vi "Write Stop Position.vi"(8 "error in (no error)":errorcluster, 10 "Stop Position":u32, 11 "Video File in":refnum<class "Video File.lvclass">) -> (0 "error out":errorcluster, 3 "Video File out":refnum<class "Video File.lvclass">)   [LabVIEW 2018, in "Video File.lvclass"]
uses:
  Video File.lvclass
  Video File.lvclass/Video File.ctl
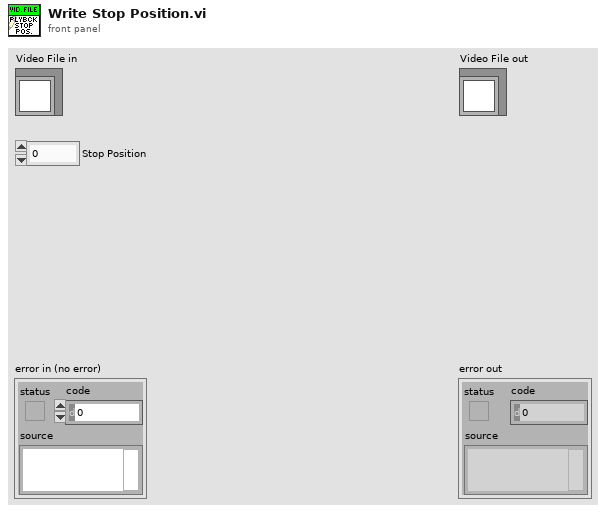
[diagram p1: front panel]
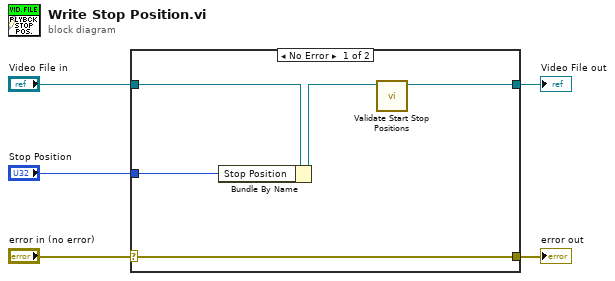
[diagram p0: block diagram]
diagram:
  n1 = case shown="No Error" "error in (no error)" {
    selector: "error in (no error)" -> [w10 w11]
    tunnel: [w10 w11] -> w4
    tunnel: [w6 w12] -> w2
    tunnel: "Video File in" -> [w9 w12]
    tunnel: "Stop Position" -> [w8 _]
    frame No Error {
      n2 = Bundle By Name(cluster=w9, "Stop Position"=w8) -> (w7:refnum<class "Video File.lvclass">)
      n3 = call-dynamic "Validate Start Stop Positions.vi"("Video File in"=w7) -> ("Video File out"=w6:refnum<class "Video File.lvclass">)  [unwired: 9 in, 1 out]
    }
    frame Error {
    }
  }
  "error out" <- w4
  "Video File out" <- w2
